vi "Wait in us.vi"(1 "Wait(us)":u64=100000 format="%.0p", 3 "Counts In":u64) -> (0 "Counts Out":u64=100)   [LabVIEW 2024]
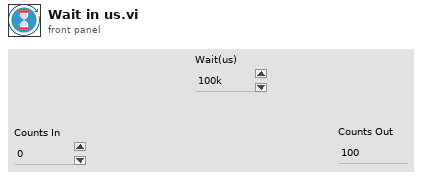
[diagram p1: front panel]
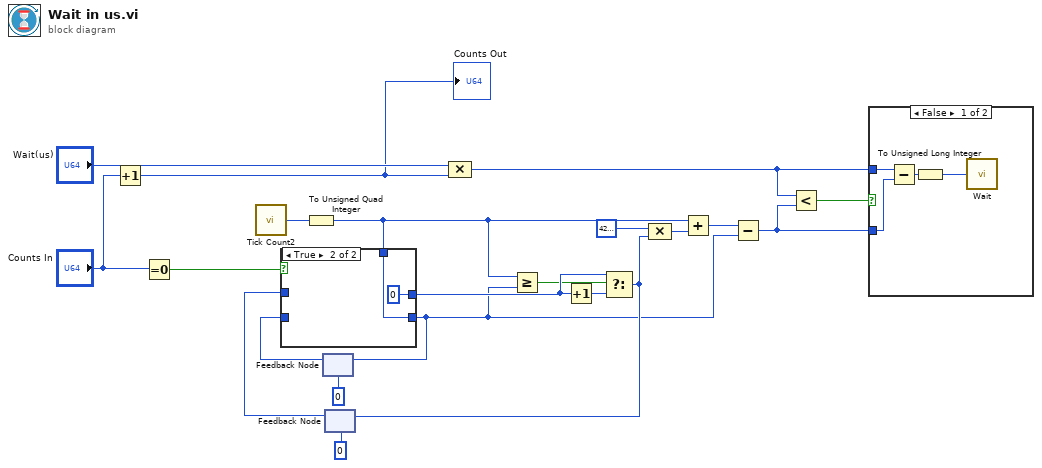
[diagram p0: block diagram]
diagram:
  n1 = Increment(x="Counts In") -> (x+1=w6:u64)
  "Counts Out" <- w6
  n2 = Equal To 0?(x="Counts In") -> (x = 0?=w8:bool)
  n3 = call "Tick Count2"() -> ("Tick Count(uSec)"=w18:u32)
  n4 = To Unsigned Quad Integer(1:w18) -> (0:w3:u64)
  n5 = feedback #1(u64 0 ("Tick Count(uSec)")) -> (w21:u64)
  n6 = feedback #2(u64 0 ("y")) -> (w5:u64)
  n7 = case shown="True" w8 {
    tunnel: [w23 w25] -> w1
    tunnel: w21 -> [w23 _]
    tunnel: w3 -> [_ w25]
    tunnel: [w22 u64 0 ("y")] -> w4
    tunnel: w5 -> [w22 _]
    frame False {
    }
    frame True {
    }
  }
  n8 = feedback-in #1(w1) -> ()
  n9 = Compound Arithmetic op=MULTIPLY("Wait(us)", w6) -> (w11:u64)
  n10 = Greater Or Equal?(x=w3, y=w1) -> (x >= y?=w2:bool)
  n11 = Increment(x=w4) -> (x+1=w17:u64)
  n12 = Select(t=w4, s=w2, f=w17) -> (s? t:f=w15:u64)
  n13 = feedback-in #2(w15) -> ()
  n14 = Compound Arithmetic op=MULTIPLY(u64 4294967295 ("y"), w15) -> (w14:u64)
  n15 = Add(x=w3, y=w14) -> (x+y=w13:u64)
  n16 = Subtract(x=w13, y=w1) -> (x-y=w10:u64)
  n17 = Less?(x=w11, y=w10) -> (x < y?=w9:bool)
  n18 = case shown="False" w9 {
    tunnel: w11 -> [w29 _]
    tunnel: w10 -> [w28 _]
    frame False {
      n19 = Subtract(x=w29, y=w28) -> (x-y=w26:u64)
      n20 = To Unsigned Long Integer(number=w26) -> (unsigned 32bit integer=w27:u32)
      n21 = call "Wait"("Count(uSec)"=w27) -> ()  [unwired: 1 out]
    }
    frame True {
    }
  }
